vi "LS-50 Send Command.vi"(0 "VISA Ref":refnum<visa-resource-name>, 2 "Read Reply?":bool=TRUE, 7 "Error In":errorcluster, 11 "Command":string) -> (4 "VISA Ref Out":refnum<visa-resource-name>, 8 "Error Out":errorcluster, 15 "Response":string)   [LabVIEW 2020]
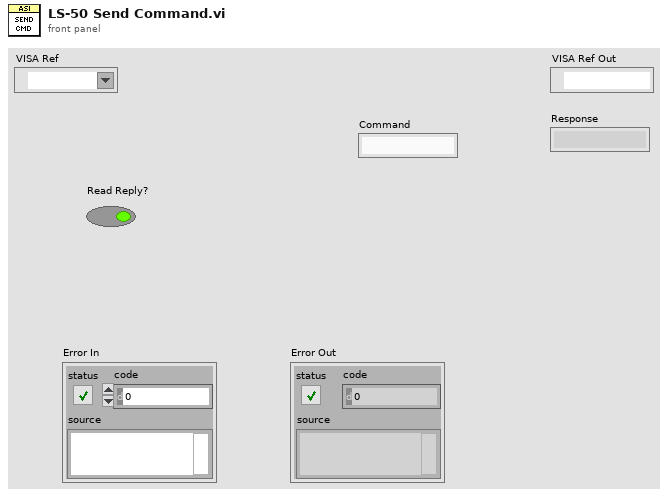
[diagram p1: front panel]
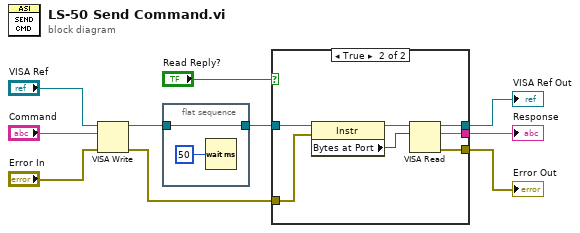
[diagram p0: block diagram]
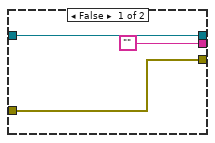
[diagram p2: hidden frame]
diagram:
  n1 = VISA Write(VISA resource name="VISA Ref", write buffer="Command", error in (no error)="Error In") -> (VISA resource name out=w3:refnum<visa-resource-name>, error out=w1:errorcluster)  [unwired: 1 out]
  n2 = flat-sequence {
    tunnel: [w11] -> w2
    tunnel: w3 -> [w11]
    frame #0 {
      n3 = Wait (ms)(milliseconds to wait=u32 50) -> ()  [unwired: 1 out]
    }
  }
  n4 = case shown="True" "Read Reply?" {
    tunnel: w2 -> [w15 w19]
    tunnel: w1 -> [w14 w18]
    tunnel: [w15 w22] -> w9
    tunnel: [w14 w21] -> w8
    tunnel: ["" w20] -> w6
    frame False {
    }
    frame True {
      n5 = property class="Instr"(reference=w19, error in=w18) -> (reference out=w16:refnum<visa-resource-name>, "Bytes at Port"=w17:u32)  [unwired: 1 out]
      n6 = VISA Read(VISA resource name=w16, byte count=w17) -> (VISA resource name out=w22:refnum<visa-resource-name>, read buffer=w20:string, error out=w21:errorcluster)  [unwired: 1 in, 1 out]
    }
  }
  "Response" <- w6
  "VISA Ref Out" <- w9
  "Error Out" <- w8
